vi "parse_range.vi"(4 "error in":errorcluster, 7 "msg in":string) -> (0 "error out":errorcluster, 1 "Header":T1, 2 "Range Data":T2, 3 "msg out":string)   [LabVIEW 2012]
doc: "Parses a message into a range"
uses:
  <userlib>/ROS for LabVIEW Software/ROS/MessageParsing/std_msgs/subs/parse_u8_scalar.vi
  <userlib>/ROS for LabVIEW Software/ROS/MessageParsing/std_msgs/subs/parse_float32_scalar.vi
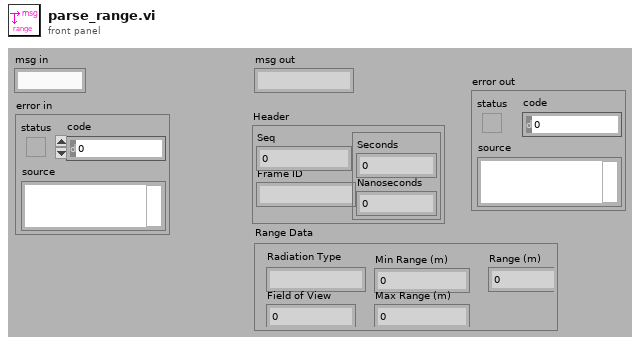
[diagram p1: front panel]
types:
  T1 = cluster{"Seq":u32, "Frame ID":string, cluster{"Seconds":i32, "Nanoseconds":i32}}
  T2 = cluster{"Radiation Type":string, "Field of View":sgl, "Min Range (m)":sgl, "Max Range (m)":sgl, "Range (m)":sgl}
  T3 = cluster{"Seq":u32, "Frame ID":string, "Timestamp":cluster{"Seconds":i32, "Nanoseconds":i32}}
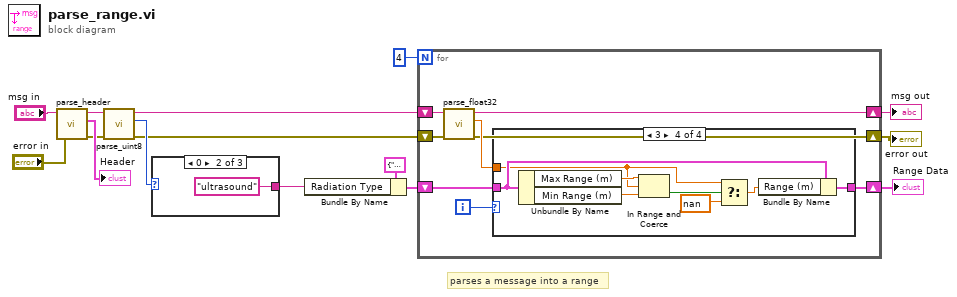
[diagram p0: block diagram]
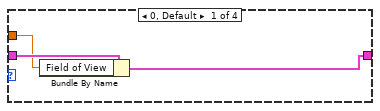
[diagram p2: hidden frame]
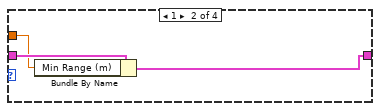
[diagram p3: hidden frame]
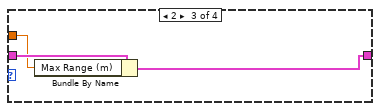
[diagram p4: hidden frame]
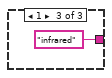
[diagram p6: hidden frame]
diagram:
  # "parses a message into a range"
  n1 = call <userlib>:"parse_header.vi"("error in"="error in", "msg in"="msg in") -> ("error out"=w3:errorcluster, "Header"=→"Header":T3, "msg out"=w14:string)  [unwired: 3 in]
  n2 = call-poly <userlib>:"parse_uint8.vi"("error in"=w3, "msg in"=w14) -> ("error out"=w2:errorcluster, "number"=w11:u8, "msg out"=w9:string)  [unwired: 3 in]
  n3 = case shown="0" w11 {
    tunnel: [_ "ultrasound" "infrared"] -> w10
    frame Default {
    }
    frame 0 {
    }
    frame 1 {
    }
  }
  n4 = Bundle By Name(cluster=T2 {"Radiation Type"="", "Field of View"=0.0, "Min Range (m)"=0.0, "Max Range (m)"=0.0, "Range (m)"=0.0} ("Range Data"), "Radiation Type"=w10) -> (w7:T2)
  n5 = for {
    N: 4 -> [_]
    shift-right: [w24] -> w5
    shift-left: w9 -> [w25]
    shift-right: [w20] -> w6
    shift-left: w7 -> [w22]
    shift-right: [w18] -> w1
    shift-left: w2 -> [w19]
    i -> [w23]
    n6 = call-poly <userlib>:"parse_float32.vi"("error in"=w19, "msg in"=w25) -> ("error out"=w18:errorcluster, "number"=w21:sgl, "msg out"=w24:string)  [unwired: 3 in]
    n7 = case shown="3" w23 {
      tunnel: w22 -> [w28 w31 w34 w41]
      tunnel: w21 -> [w27 w29 w32 w36]
      tunnel: [w26 w30 w33 w42] -> w20
      frame 0, Default {
        n8 = Bundle By Name(cluster=w28, "Field of View"=w27) -> (w26:T2)
      }
      frame 1 {
        n9 = Bundle By Name(cluster=w31, "Min Range (m)"=w29) -> (w30:T2)
      }
      frame 2 {
        n10 = Bundle By Name(cluster=w34, "Max Range (m)"=w32) -> (w33:T2)
      }
      frame 3 {
        n11 = Unbundle By Name(w41) -> ("Max Range (m)"=w38:sgl, "Min Range (m)"=w37:sgl)
        n12 = In Range and Coerce(upper limit=w38, x=w36, lower limit=w37) -> (In Range?=w40:bool)  [unwired: 1 out]
        n13 = Select(t=w36, s=w40, f=sgl nan) -> (s? t:f=w35:sgl)
        n14 = Bundle By Name(cluster=w41, "Range (m)"=w35) -> (w42:T2)
      }
    }
  }
  "Range Data" <- w6
  "msg out" <- w5
  "error out" <- w1
